vi "FPGA.vi"() -> ()   [LabVIEW 2016]
uses:
  <vilib>/EmbeddedDisplay/Hitachi HD44780/Common/Control/lcd command cluster.ctl
  <vilib>/Platform/TimedLoop/XDataNode/timing_clust.ctl
  <vilib>/Platform/TimedLoop/XDataNode/nitl_modes.ctl
  <vilib>/Platform/TimedLoop/XDataNode/wakeup.ctl
  <vilib>/EmbeddedDisplay/Hitachi HD44780/Common/Control/8bit connection map.ctl
  <vilib>/rvi/Emulation/niFpgaGetClockAttributes.vi
  <vilib>/rvi/Emulation/niFpgaSctlEmulationGetInTimedLoop.vi
  <vilib>/rvi/Emulation/niFpgaEmulationReportErrorSimple.vi
  <vilib>/rvi/Emulation/niFpgaProcessEmulError.vi
  <vilib>/EmbeddedDisplay/Hitachi HD44780/FPGA/Internal/LCD Command.vi
  <vilib>/EmbeddedDisplay/Hitachi HD44780/FPGA/Public/Command Handler (8 Bits).vi
  <vilib>/rvi/Emulation/niFpgaCriticalErrorInLSC.vi
  <vilib>/rvi/interface/RandomDataEmulation/niFpgaRandomDataHandleErrors.vi
  <vilib>/rvi/eio/common/nirviEmuTemplateMethod_errors.vi
  <vilib>/rvi/DataTransferAndStorage/Container/XNode/niFpgaContainer.xnode
  <vilib>/rvi/interface/RandomDataEmulation/nirviRandomDataFpgaReadWriteTemplate.vi
  <vilib>/eio/EIONode/EIONode.xnode
  <vilib>/Platform/TimedLoop/XDataNode/XDataNode.xnode
  <vilib>/EmbeddedDisplay/Hitachi HD44780/Common/HD44780 Common.lvlib
  <vilib>/EmbeddedDisplay/Hitachi HD44780/FPGA/HD44780 FPGA.lvlib
  <vilib>/Platform/TimedLoop/XDataNode/XDNodeRunTimeDep.lvlib
panel:
  in  "Gain":fxp<+/-,32,16> format="%.21g"
  out "E-Stop":bool
  in  "PWM":bool
  out "Position":i16
  in  "Reset":bool
  in  "LCD Command":T1={"device index (-1)"=-1, "operation (0)"=0}
  # "Encoder Loop"
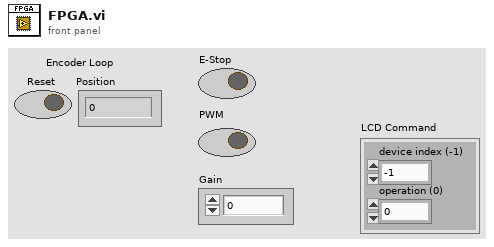
[diagram p1: front panel]
types:
  T1 = typedef "HD44780 Common.lvlib/lcd command cluster.ctl" = cluster{"device index (-1)":i8, "operation (0)":u32}
  T2 = typedef "XDNodeRunTimeDep.lvlib/timing_clust.ctl" = cluster{"Expected End [f-1]":u64, "Actual End [f-1]":u64, "Finished Late? [f-1]":bool, "Expected End [i-1]":u64, "Actual End [i-1]":u64, "Finished Late? [i-1]":bool, "Expected Start [i]":u64, "Actual Start [i]":u64, "Expected Start [f]":u64, "Actual Start [f]":u64, "Source Name":string, "Structure Name":string, "Period":i64, "Deadline":i64, "Offset":i64, "Start":i64, "Priority":i32, "Timeout":i32, "Mode":T3, "Wakeup Reason":T4, "Error":errorcluster, "Source Type":string, "Secondary Source Type":string, "Global End Time":u64, "Global Start Time":u64, "Frame Duration":u64, "Iteration Duration":u64, "Assigned CPU":i32, "I/O Scan Engine Mode":u32}
  T3 = typedef "XDNodeRunTimeDep.lvlib/nitl_modes.ctl" = enum32{"No Change", "Process missed periods, maintain original phase", "Discard missed periods, maintain original phase", "Process missed periods, ignore original phase", "Discard missed periods, ignore original phase"}
  T4 = typedef "XDNodeRunTimeDep.lvlib/wakeup.ctl" = enum32{"Normal", "Aborted", "Asynchronous wakeup", "Timing source error", "Timed loop error", "Timeout"}
  T5 = typedef "HD44780 Common.lvlib/8bit connection map.ctl" = cluster{"RS":refnum<k21>, "R/W":refnum<k21>, "E1":refnum<k21>, "E2":refnum<k21>, "DB0":refnum<k21>, "DB1":refnum<k21>, "DB2":refnum<k21>, "DB3":refnum<k21>, "DB4":refnum<k21>, "DB5":refnum<k21>, "DB6":refnum<k21>, "DB7":refnum<k21>}
  T6 = cluster{"device index (-1)":i8, "operation (0)":u32}
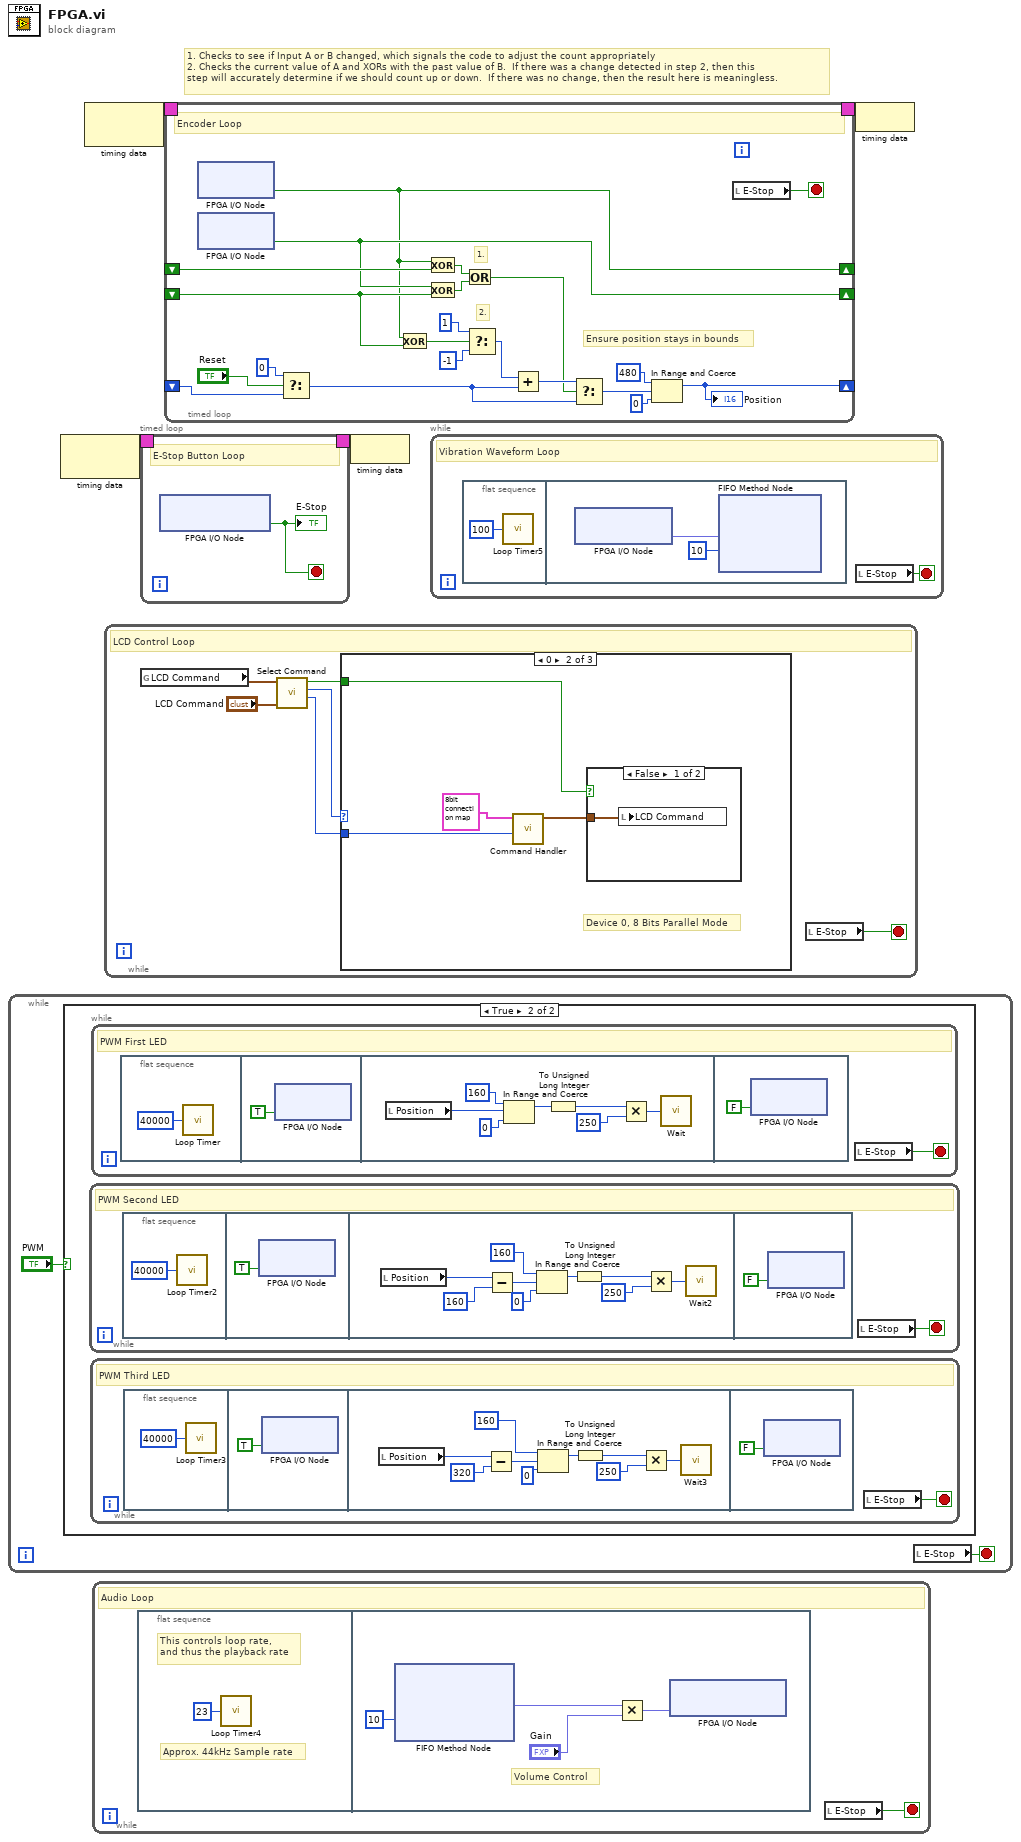
[diagram p0: block diagram]
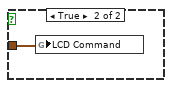
[diagram p3: hidden frame]
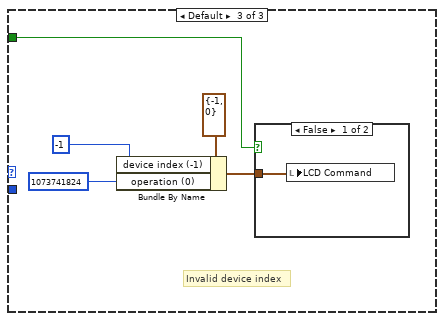
[diagram p4: hidden frame]
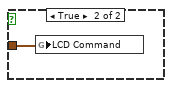
[diagram p5: hidden frame]
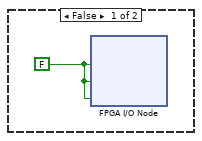
[diagram p6: hidden frame]
diagram:
  # "1. Checks to see if Input A or B changed, which signals the code to adjust the count appropriately\n2. Checks the current value of A and XORs with the past value of B.  If there was a change detected in step 2, then this \nstep will accurately determine if we should count up or down.  If there was no change, then the result here is meaningless."
  n1 = while {
    stop <- w5 stop-if-true
    n2 = case shown="True" "PWM" {
      frame False {
        w7 = FALSE ("DIO4")
        n3 = xnode "FPGA I/O Node"("LED1"=w7, "LED2"=w7, "LED3"=w7) -> ()  [unwired: 3 in, 3 out]
      }
      frame True {
        n4 = while {
          stop <- w21 stop-if-true
          # "PWM Second LED"
          n5 = flat-sequence {
            frame #0 {
              n6 = call "Loop Timer2"("Count(Ticks)"=u32 40000) -> ()  [unwired: 1 out]
            }
            frame #1 {
              n7 = xnode "FPGA I/O Node"("LED2"=TRUE ("DIO5")) -> ()  [unwired: 1 in, 1 out]
            }
            frame #2 {
              n8 = local read "Position"() -> (w26:i16)
              n9 = Subtract(x=w26, y=i16 160) -> (x-y=w28:i16)
              n10 = In Range and Coerce(upper limit=i16 160, x=w28, lower limit=i16 0) -> (coerced(x)=w25:i16)  [unwired: 1 out]
              n11 = To Unsigned Long Integer(number=w25) -> (unsigned 32bit integer=w24:u32)
              n12 = Multiply(x=w24, y=u32 250) -> (x*y=w29:u32)
              n13 = call "Wait2"("Count(Ticks)"=w29) -> ()  [unwired: 1 out]
            }
            frame #3 {
              n14 = xnode "FPGA I/O Node"("LED2"=FALSE ("DIO5")) -> ()  [unwired: 1 in, 1 out]
            }
          }
          n15 = local read "E-Stop"() -> (w21:bool)
        }
        n16 = while {
          stop <- w8 stop-if-true
          # "PWM Third LED"
          n17 = flat-sequence {
            frame #0 {
              n18 = call "Loop Timer3"("Count(Ticks)"=u32 40000) -> ()  [unwired: 1 out]
            }
            frame #1 {
              n19 = xnode "FPGA I/O Node"("LED3"=TRUE ("DIO5")) -> ()  [unwired: 1 in, 1 out]
            }
            frame #2 {
              n20 = local read "Position"() -> (w13:i16)
              n21 = Subtract(x=w13, y=i16 320) -> (x-y=w14:i16)
              n22 = In Range and Coerce(upper limit=i16 160, x=w14, lower limit=i16 0) -> (coerced(x)=w12:i16)  [unwired: 1 out]
              n23 = To Unsigned Long Integer(number=w12) -> (unsigned 32bit integer=w11:u32)
              n24 = Multiply(x=w11, y=u32 250) -> (x*y=w16:u32)
              n25 = call "Wait3"("Count(Ticks)"=w16) -> ()  [unwired: 1 out]
            }
            frame #3 {
              n26 = xnode "FPGA I/O Node"("LED3"=FALSE ("DIO5")) -> ()  [unwired: 1 in, 1 out]
            }
          }
          n27 = local read "E-Stop"() -> (w8:bool)
        }
        n28 = while {
          stop <- w34 stop-if-true
          # "PWM First LED"
          n29 = flat-sequence {
            frame #0 {
              n30 = call "Loop Timer"("Count(Ticks)"=u32 40000) -> ()  [unwired: 1 out]
            }
            frame #1 {
              n31 = xnode "FPGA I/O Node"("LED1"=TRUE ("DIO5")) -> ()  [unwired: 1 in, 1 out]
            }
            frame #2 {
              n32 = local read "Position"() -> (w39:i16)
              n33 = In Range and Coerce(upper limit=i16 160, x=w39, lower limit=i16 0) -> (coerced(x)=w38:i16)  [unwired: 1 out]
              n34 = To Unsigned Long Integer(number=w38) -> (unsigned 32bit integer=w37:u32)
              n35 = Multiply(x=w37, y=u32 250) -> (x*y=w40:u32)
              n36 = call "Wait"("Count(Ticks)"=w40) -> ()  [unwired: 1 out]
            }
            frame #3 {
              n37 = xnode "FPGA I/O Node"("LED1"=FALSE ("DIO5")) -> ()  [unwired: 1 in, 1 out]
            }
          }
          n38 = local read "E-Stop"() -> (w34:bool)
        }
      }
    }
    n39 = local read "E-Stop"() -> (w5:bool)
  }
  n40 = node-c288() -> (w2:T2)  [unwired: 1 in]
  n41 = node-c288() -> (w4:T2)  [unwired: 1 in]
  n42 = while {
    stop <- w45 stop-if-true
    # "Audio Loop"
    n43 = flat-sequence {
      frame #0 {
        # "Approx. 44kHz Sample rate"
        # "This controls loop rate,\nand thus the playback rate"
        n44 = call "Loop Timer4"("Count(uSec)"=u32 23) -> ()  [unwired: 1 out]
      }
      frame #1 {
        # "Volume Control"
        n45 = xnode ("FIFO Method Node")("Timeout"=10) -> ("Element"=w48:fxp<+/-,32,16>)  [unwired: 1 in, 2 out]
        n46 = Multiply(x=w48, y="Gain") -> (x*y=w49:fxp<+/-,64,32>)
        n47 = xnode "FPGA I/O Node"("Audio Output"=w49) -> ()  [unwired: 1 in, 1 out]
      }
    }
    n48 = local read "E-Stop"() -> (w45:bool)
  }
  n49 = while {
    stop <- w51 stop-if-true
    # "LCD Control Loop"
    n50 = global read "LCD Command.vi" "LCD Command"() -> (w52:T6)
    n51 = call <vilib>:"Select Command.vi"("Host LCD Command"="LCD Command", "FPGA LCD Command"=w52) -> ("operation"=w54:u32, "device index"=w55:i8, "FPGA? True : False"=w53:bool)  [unwired: 7 in]
    n52 = case shown="0" w55 {
      tunnel: w54 -> [_ w60 _]
      tunnel: w53 -> [_ w59 w67]
      frame -1 {
        # "IDLE State"
      }
      frame 0 {
        # "Device 0, 8 Bits Parallel Mode"
        n53 = call-poly <vilib>:"Command Handler.vi"("operation"=w60, "device connection map in"=T5 {"RS"="DIO19", "R/W"="DIO18", "E1"="DIO17", "E2"="DIO17", "DB0"="DIO20", "DB1"="DIO21", "DB2"="DIO22", "DB3"="DIO23", "DB4"="DIO24", "DB5"="DIO25", "DB6"="DIO26", "DB7"="DIO27"}) -> ("result"=w58:T6)  [unwired: 9 in]
        n54 = case shown="False" w59 {
          tunnel: w58 -> [w61 w62]
          frame False {
            n55 = local write "LCD Command"(w61) -> ()
          }
          frame True {
            n56 = global write "LCD Command.vi" "LCD Command"(w62) -> ()
          }
        }
      }
      frame Default {
        # "Invalid device index"
        n57 = Bundle By Name(cluster=T1 {"device index (-1)"=-1, "operation (0)"=0} ("LCD Command"), "device index (-1)"=i8 -1 ("LCD_device index (-1)"), "operation (0)"=u32 1073741824 ("LCD_operation (0)")) -> (w63:T1)
        n58 = case shown="False" w67 {
          tunnel: w63 -> [w68 w69]
          frame False {
            n59 = local write "LCD Command"(w68) -> ()
          }
          frame True {
            n60 = global write "LCD Command.vi" "LCD Command"(w69) -> ()
          }
        }
      }
    }
    n61 = local read "E-Stop"() -> (w51:bool)
  }
  n62 = timed-loop {
    timing: w2 -> [_]
    timing-out: [_] -> w1
    stop <- w70 stop-if-true
    # "E-Stop Button Loop"
    n63 = xnode "FPGA I/O Node"() -> ("Right Button"=w70:bool)  [unwired: 1 in, 1 out]
    "E-Stop" <- w70
  }
  n64 = timed-loop {
    shift-left: _ -> [w81]
    shift-right: [w80] -> _
    shift-left: _ -> [w90]
    shift-right: [w78] -> _
    shift-left: _ -> [w86]
    shift-right: [w73] -> _
    timing: w4 -> [_]
    timing-out: [_] -> w3
    stop <- w74 stop-if-true
    # "2."
    # "1."
    # "Ensure position stays in bounds"
    # "Encoder Loop"
    n65 = xnode "FPGA I/O Node"() -> ("DIO10"=w73:bool)  [unwired: 1 in, 1 out]
    n66 = xnode "FPGA I/O Node"() -> ("DIO11"=w80:bool)  [unwired: 1 in, 1 out]
    n67 = Select(t=i16 0, s="Reset", f=w90) -> (s? t:f=w91:i16)
    n68 = Exclusive Or(1:w81, 2:w73) -> (0:w82:bool)
    n69 = Exclusive Or(1:w86, 2:w73) -> (0:w84:bool)
    n70 = Exclusive Or(1:w81, 2:w80) -> (0:w85:bool)
    n71 = Or(x=w84, y=w85) -> (x .or. y?=w83:bool)
    n72 = Select(t=i16 1, s=w82, f=i16 -1) -> (s? t:f=w89:i16)
    n73 = Add(x=w89, y=w91) -> (x+y=w93:i16)
    n74 = Select(t=w93, s=w83, f=w91) -> (s? t:f=w79:i16)
    n75 = In Range and Coerce(upper limit=i16 480, x=w79, lower limit=i16 0) -> (coerced(x)=w78:i16)  [unwired: 1 out]
    "Position" <- w78
    n76 = local read "E-Stop"() -> (w74:bool)
  }
  n77 = node-c288(w1) -> ()
  n78 = while {
    stop <- w96 stop-if-true
    # "Vibration Waveform Loop"
    n79 = flat-sequence {
      frame #0 {
        n80 = call "Loop Timer5"("Count(uSec)"=u32 100) -> ()  [unwired: 1 out]
      }
      frame #1 {
        n81 = xnode "FPGA I/O Node"() -> ("Sine Wave"=w98:fxp<+/-,24,5>)  [unwired: 1 in, 1 out]
        n82 = xnode ("FIFO Method Node")("Element"=w98, "Timeout"=10) -> ()  [unwired: 1 in, 2 out]
      }
    }
    n83 = local read "E-Stop"() -> (w96:bool)
  }
  n84 = node-c288(w3) -> ()
